vi "4_Byte_to_SGL.vi"(0 "Array of 4 bytes":u8[](array[numeric]) format="%.0x", 1 "number of valid bytes":u8) -> (2 "Status Code":i16, 3 "Number":sgl format="%.4f")   [LabVIEW 2017]
doc: "Convert 4 byte float to a SGL numeric. Conversion is done according to IEEE 754-1990."
panel:
  # "Convert array of singleprecision float to SGL value (IEEE 754-1990)\nC.Holmstedt 2002-03-06\nAdded check for status byte at end per FEMC ICD.\nM.McLeod 2006-08-02"
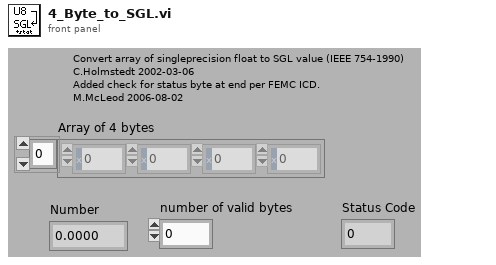
[diagram p1: front panel]
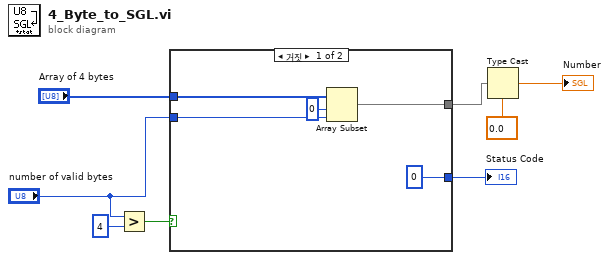
[diagram p0: block diagram]
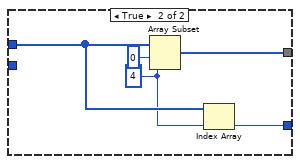
[diagram p2: hidden frame]
diagram:
  n1 = Greater?(x="number of valid bytes", y=u8 4) -> (0:w5:bool)
  n2 = case shown="거짓" w5 {
    tunnel: [u8 0 w18] -> w1
    tunnel: "number of valid bytes" -> [w12 _]
    tunnel: "Array of 4 bytes" -> [w11 w15]
    tunnel: [w10 w16] -> w2
    frame False {
      n3 = Array Subset(array=w11, index=0 ("Array Index"), length=w12) -> (w10:u8[])
    }
    frame True {
      w14 = 4 ("length")
      n4 = Array Subset(array=w15, index=0 ("Array Index"), length=w14) -> (w16:u8[])
      n5 = Index Array(array=w15, index=w14) -> (element=w18:u8)
    }
  }
  "Status Code" <- w1
  n6 = Type Cast(type=sgl 0.0, x=w2) -> (*(type *) &x=→"Number":sgl)
